vi "WPI_CANJaguar_GetPID.vi"(0 "CAN Jaguar Ref":T1={"DeviceStatus"={"status"=FALSE, "code"=0, "source"=""}, "Type"=enum."PWM", "PWM"={"PWM Channel"=enum."PWM 1", "DeadBand"={"Name"="", "maxPositivePwm"=0, "minPositivePwm"=0, "centerPwm"=0, "maxNegativePwm"=0, "minNegativePwm"=0, "angularRange"=0}}, "CAN"={"Device Number"=0, "SetOutput VI Ref"=variant(enum8{"Percent VBus", "Current", "Speed", "Position", "Voltage"} enum."Percent VBus"), "GetOutput VI Ref"=variant(refnum<k1> refnum), "Enable VI Ref"=variant(dbl 12.0), "Disable VI Ref"=variant(enum8{"Percent VBus", "Speed", "Position", "Slave", "Unchanged / Invalid", "Voltage Compensation", "Current", "Motion Profile"} enum."Percent VBus"), "Data"=variant}, "Invert"=FALSE}, 11 "error in (no error)":errorcluster) -> (4 "CAN Jaguar Ref":T1={"DeviceStatus"={"status"=FALSE, "code"=0, "source"=""}, "Type"=enum."PWM", "PWM"={"PWM Channel"=enum."PWM 1", "DeadBand"={"Name"="", "maxPositivePwm"=0, "minPositivePwm"=0, "centerPwm"=0, "maxNegativePwm"=0, "minNegativePwm"=0, "angularRange"=0}}, "CAN"={"Device Number"=0, "SetOutput VI Ref"=variant(enum8{"Percent VBus", "Current", "Speed", "Position", "Voltage"} enum."Percent VBus"), "GetOutput VI Ref"=variant(refnum<k1> refnum), "Enable VI Ref"=variant(dbl 12.0), "Disable VI Ref"=variant(enum8{"Percent VBus", "Speed", "Position", "Slave", "Unchanged / Invalid", "Voltage Compensation", "Current", "Motion Profile"} enum."Percent VBus"), "Data"=variant}, "Invert"=FALSE}, 6 "P":dbl, 8 "I":dbl, 10 "D":dbl, 15 "error out":errorcluster)   [LabVIEW 2016]
doc: "Get the PID constants that are being used by the active controller on the Jaguar.\n\nThis VI only applies in <B>Current</B>, <B>Position</B>, and <B>Speed</B> modes."
uses:
  <vilib>/Rock Robotics/WPI/MotorControl/WPI_MotorControlDeviceRef.ctl
  <vilib>/Rock Robotics/WPI/MotorControl/WPI_MotorControlType.ctl
  <vilib>/Rock Robotics/SystemInterfaces/DIO/FPGA_DIOPWMChannel.ctl
  <vilib>/Rock Robotics/WPI/PWM/WPI_PWMDeadband.ctl
  <vilib>/Rock Robotics/WPI/ThirdParty/CanMotor/CAN Jaguar/SubVIs/WPI_CANJaguar_RefNumData.ctl
  <vilib>/Rock Robotics/WPI/ThirdParty/CanMotor/CAN Jaguar/SubVIs/WPI_CANJaguar_ControlMode.ctl
  <vilib>/Rock Robotics/WPI/ThirdParty/CanMotor/CAN Jaguar/SubVIs/WPI_CAN_MotorMessageIDs.ctl
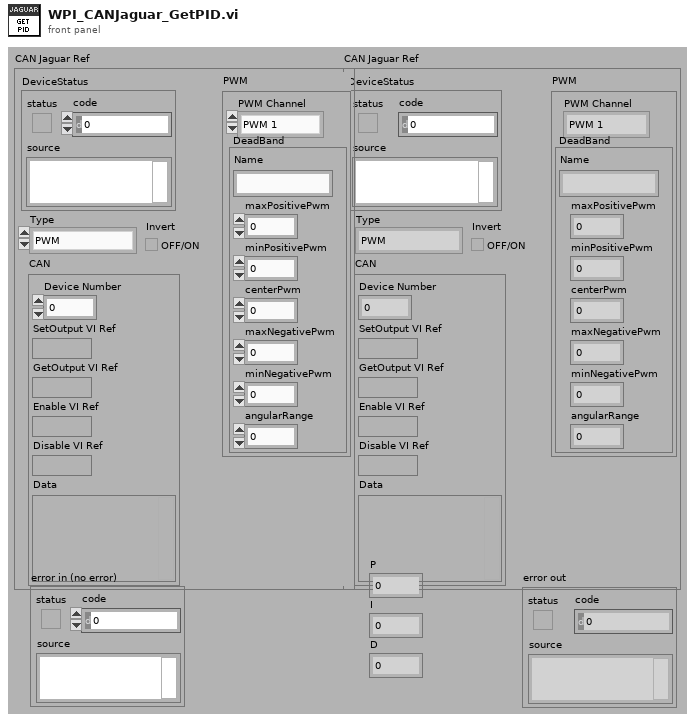
[diagram p1: front panel]
types:
  T1 = typedef "WPI_MotorControlDeviceRef.ctl" = cluster{"DeviceStatus":errorcluster, "Type":T2, "PWM":cluster{"PWM Channel":T3, "DeadBand":T4}, "CAN":cluster{"Device Number":u8, "SetOutput VI Ref":variant, "GetOutput VI Ref":variant, "Enable VI Ref":variant, "Disable VI Ref":variant, "Data":variant}, "Invert":bool}
  T2 = typedef "WPI_MotorControlType.ctl" = enum16{"PWM", "CAN"}
  T3 = typedef "FPGA_DIOPWMChannel.ctl" = enum8{"PWM 0", "PWM 1", "PWM 2", "PWM 3", "PWM 4", "PWM 5", "PWM 6", "PWM 7", "PWM 8", "PWM 9", "PWM MXP 0", "PWM MXP 1", "PWM MXP 2", "PWM MXP 3", "PWM MXP 4", "PWM MXP 5", "PWM MXP 6", "PWM MXP 7", "PWM MXP 8", "PWM MXP 9", "Invalid"}
  T4 = typedef "WPI_PWMDeadband.ctl" = cluster{"Name":string, "maxPositivePwm":i32, "minPositivePwm":i32, "centerPwm":i32, "maxNegativePwm":i32, "minNegativePwm":i32, "angularRange":u16}
  T5 = typedef "WPI_CANJaguar_RefNumData.ctl" = cluster{"CAN.Max Vout":dbl, "Control Mode":T6, "semaphore":T7}
  T6 = typedef "WPI_CANJaguar_ControlMode.ctl" = enum8{"Percent VBus", "Current", "Speed", "Position", "Voltage"}
  T7 = typedef "Semaphore RefNum" = refnum<k1>
  T8 = typedef "WPI_CAN_MotorMessageIDs.ctl" = u32
  T9 = enum16{"big-endian, network order", "native, host order", "little-endian"}
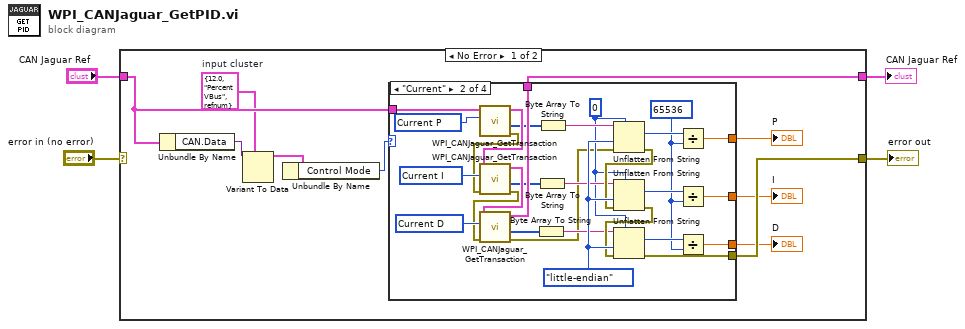
[diagram p0: block diagram]
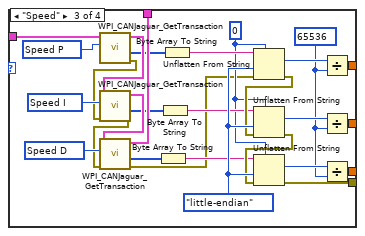
[diagram p3: hidden frame]
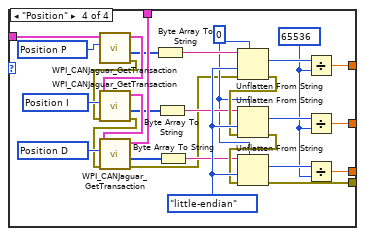
[diagram p4: hidden frame]
diagram:
  n1 = case shown="No Error" "error in (no error)" {
    selector: "error in (no error)" -> [_ w100]
    tunnel: [w9 w101] -> w4
    tunnel: "CAN Jaguar Ref" -> [w10 w101]
    tunnel: [w14 w100] -> w2
    frame No Error {
      w7 = T5 {"CAN.Max Vout"=12.0, "Control Mode"=enum."Percent VBus", "semaphore"=refnum}  # input cluster
      n2 = Unbundle By Name(w10) -> ("CAN.Data"=w8:variant)
      n3 = Variant To Data(type=w7, Variant=w8) -> (data=w6:T5)  [unwired: 1 in, 1 out]
      n4 = Unbundle By Name(w6) -> ("Control Mode"=w5:T6)
      n5 = case shown="\"Current\"" w5 {
        tunnel: [_ w34 w62 w90] -> w13
        tunnel: [_ w36 w64 w92] -> w14
        tunnel: [_ w32 w60 w88] -> w12
        tunnel: [_ w30 w58 w86] -> w11
        tunnel: w10 -> [w15 w28 w56 w84]
        tunnel: [w15 w21 w50 w78] -> w9
        frame Default {
        }
        frame "Current" {
          w29 = 65536 ("y")
          w26 = T8 33689856 items=["Volt Enable"=33685504, "Volt Disable"=33685568, "Volt Set"=33685632, "Volt Set Ramp"=33685696, "Speed Enable"=33686528, "Speed Disable"=33686592, "Speed Set"=33686656, "Speed P"=33686720, "Speed I"=33686784, "Speed D"=33686848, "Speed Ref"=33686912, "Volt Comp Enable"=33687552, "Volt Comp Disable"=33687616, "Volt Comp Set"=33687680, "Volt Comp In Ramp"=33687744, "Volt Comp Comp Ramp"=33687808, "Position Enable"=33688576, "Position Disable"=33688640, "Position Set"=33688704, "Position P"=33688768, "Position I"=33688832, "Position D"=33688896, "Position Ref"=33688960, "Current Enable"=33689600, "Current Disable"=33689664, "Current Set"=33689728, "Current P"=33689792, "Current I"=33689856, "Current D"=33689920, "Status Percent VBus"=33690624, "Status VBus"=33690688, "Status Current"=33690752, "Status Temp"=33690816, "Status Position"=33690880, "Status Speed"=33690944, "Status Limit"=33691008, "Status Fault"=33691072, "Status Power"=33691136, "Status Control Mode"=33691200, "Status VOut"=33691264, "Config Num Brushes"=33692672, "Config Encoder Lines"=33692736, "Config Pot Turns"=33692800, "Config Brake Coast"=33692864, "Config Limit Mode"=33692928, "Config Limit Fwd"=33692992, "Config Limit Rev"=33693056, "Config Max VOut"=33693120, "Config Fault Time"=33693184, "Motor Ack"=33693696] ("CAN Motor Message IDs")
          w24 = T8 33689920 items=["Volt Enable"=33685504, "Volt Disable"=33685568, "Volt Set"=33685632, "Volt Set Ramp"=33685696, "Speed Enable"=33686528, "Speed Disable"=33686592, "Speed Set"=33686656, "Speed P"=33686720, "Speed I"=33686784, "Speed D"=33686848, "Speed Ref"=33686912, "Volt Comp Enable"=33687552, "Volt Comp Disable"=33687616, "Volt Comp Set"=33687680, "Volt Comp In Ramp"=33687744, "Volt Comp Comp Ramp"=33687808, "Position Enable"=33688576, "Position Disable"=33688640, "Position Set"=33688704, "Position P"=33688768, "Position I"=33688832, "Position D"=33688896, "Position Ref"=33688960, "Current Enable"=33689600, "Current Disable"=33689664, "Current Set"=33689728, "Current P"=33689792, "Current I"=33689856, "Current D"=33689920, "Status Percent VBus"=33690624, "Status VBus"=33690688, "Status Current"=33690752, "Status Temp"=33690816, "Status Position"=33690880, "Status Speed"=33690944, "Status Limit"=33691008, "Status Fault"=33691072, "Status Power"=33691136, "Status Control Mode"=33691200, "Status VOut"=33691264, "Config Num Brushes"=33692672, "Config Encoder Lines"=33692736, "Config Pot Turns"=33692800, "Config Brake Coast"=33692864, "Config Limit Mode"=33692928, "Config Limit Fwd"=33692992, "Config Limit Rev"=33693056, "Config Max VOut"=33693120, "Config Fault Time"=33693184, "Motor Ack"=33693696] ("CAN Motor Message IDs")
          w37 = 0 ("Voltage")
          w27 = T8 33689792 items=["Volt Enable"=33685504, "Volt Disable"=33685568, "Volt Set"=33685632, "Volt Set Ramp"=33685696, "Speed Enable"=33686528, "Speed Disable"=33686592, "Speed Set"=33686656, "Speed P"=33686720, "Speed I"=33686784, "Speed D"=33686848, "Speed Ref"=33686912, "Volt Comp Enable"=33687552, "Volt Comp Disable"=33687616, "Volt Comp Set"=33687680, "Volt Comp In Ramp"=33687744, "Volt Comp Comp Ramp"=33687808, "Position Enable"=33688576, "Position Disable"=33688640, "Position Set"=33688704, "Position P"=33688768, "Position I"=33688832, "Position D"=33688896, "Position Ref"=33688960, "Current Enable"=33689600, "Current Disable"=33689664, "Current Set"=33689728, "Current P"=33689792, "Current I"=33689856, "Current D"=33689920, "Status Percent VBus"=33690624, "Status VBus"=33690688, "Status Current"=33690752, "Status Temp"=33690816, "Status Position"=33690880, "Status Speed"=33690944, "Status Limit"=33691008, "Status Fault"=33691072, "Status Power"=33691136, "Status Control Mode"=33691200, "Status VOut"=33691264, "Config Num Brushes"=33692672, "Config Encoder Lines"=33692736, "Config Pot Turns"=33692800, "Config Brake Coast"=33692864, "Config Limit Mode"=33692928, "Config Limit Fwd"=33692992, "Config Limit Rev"=33693056, "Config Max VOut"=33693120, "Config Fault Time"=33693184, "Motor Ack"=33693696] ("CAN Motor Message IDs")
          w42 = T9."little-endian" ("byte order (0:big-endian, network order)")
          n6 = call <vilib>:"WPI_CANJaguar_GetTransaction.vi"("Message ID"=w27, "CAN Jaguar Ref"=w28) -> ("error out"=w17:errorcluster, "Data Out"=w18:u8[], "CAN Jaguar Ref Out"=w25:T1)  [unwired: 1 in, 6 out]
          n7 = call <vilib>:"WPI_CANJaguar_GetTransaction.vi"("error in"=w17, "Message ID"=w26, "CAN Jaguar Ref"=w25) -> ("error out"=w16:errorcluster, "Data Out"=w19:u8[], "CAN Jaguar Ref Out"=w23:T1)  [unwired: 6 out]
          n8 = call <vilib>:"WPI_CANJaguar_GetTransaction.vi"("error in"=w16, "Message ID"=w24, "CAN Jaguar Ref"=w23) -> ("error out"=w22:errorcluster, "Data Out"=w20:u8[], "CAN Jaguar Ref Out"=w21:T1)  [unwired: 6 out]
          n9 = Byte Array To String(unsigned byte array=w20) -> (string=w38:string)
          n10 = Byte Array To String(unsigned byte array=w19) -> (string=w39:string)
          n11 = Byte Array To String(unsigned byte array=w18) -> (string=w43:string)
          n12 = Unflatten From String(type=w37, binary string=w43, byte order (0:big-endian, network order)=w42, error in (no error)=w22) -> (value=w35:i32, error out=w40:errorcluster)  [unwired: 2 out]
          n13 = Unflatten From String(type=w37, binary string=w39, byte order (0:big-endian, network order)=w42, error in (no error)=w40) -> (value=w33:i32, error out=w41:errorcluster)  [unwired: 2 out]
          n14 = Unflatten From String(type=w37, binary string=w38, byte order (0:big-endian, network order)=w42, error in (no error)=w41) -> (value=w31:i32, error out=w36:errorcluster)  [unwired: 2 out]
          n15 = Divide(x=w35, y=w29) -> (x/y=w34:dbl)
          n16 = Divide(x=w33, y=w29) -> (x/y=w32:dbl)
          n17 = Divide(x=w31, y=w29) -> (x/y=w30:dbl)
        }
        frame "Speed" {
          w57 = 65536 ("y")
          w54 = T8 33686784 items=["Volt Enable"=33685504, "Volt Disable"=33685568, "Volt Set"=33685632, "Volt Set Ramp"=33685696, "Speed Enable"=33686528, "Speed Disable"=33686592, "Speed Set"=33686656, "Speed P"=33686720, "Speed I"=33686784, "Speed D"=33686848, "Speed Ref"=33686912, "Volt Comp Enable"=33687552, "Volt Comp Disable"=33687616, "Volt Comp Set"=33687680, "Volt Comp In Ramp"=33687744, "Volt Comp Comp Ramp"=33687808, "Position Enable"=33688576, "Position Disable"=33688640, "Position Set"=33688704, "Position P"=33688768, "Position I"=33688832, "Position D"=33688896, "Position Ref"=33688960, "Current Enable"=33689600, "Current Disable"=33689664, "Current Set"=33689728, "Current P"=33689792, "Current I"=33689856, "Current D"=33689920, "Status Percent VBus"=33690624, "Status VBus"=33690688, "Status Current"=33690752, "Status Temp"=33690816, "Status Position"=33690880, "Status Speed"=33690944, "Status Limit"=33691008, "Status Fault"=33691072, "Status Power"=33691136, "Status Control Mode"=33691200, "Status VOut"=33691264, "Config Num Brushes"=33692672, "Config Encoder Lines"=33692736, "Config Pot Turns"=33692800, "Config Brake Coast"=33692864, "Config Limit Mode"=33692928, "Config Limit Fwd"=33692992, "Config Limit Rev"=33693056, "Config Max VOut"=33693120, "Config Fault Time"=33693184, "Motor Ack"=33693696] ("CAN Motor Message IDs")
          w51 = T8 33686848 items=["Volt Enable"=33685504, "Volt Disable"=33685568, "Volt Set"=33685632, "Volt Set Ramp"=33685696, "Speed Enable"=33686528, "Speed Disable"=33686592, "Speed Set"=33686656, "Speed P"=33686720, "Speed I"=33686784, "Speed D"=33686848, "Speed Ref"=33686912, "Volt Comp Enable"=33687552, "Volt Comp Disable"=33687616, "Volt Comp Set"=33687680, "Volt Comp In Ramp"=33687744, "Volt Comp Comp Ramp"=33687808, "Position Enable"=33688576, "Position Disable"=33688640, "Position Set"=33688704, "Position P"=33688768, "Position I"=33688832, "Position D"=33688896, "Position Ref"=33688960, "Current Enable"=33689600, "Current Disable"=33689664, "Current Set"=33689728, "Current P"=33689792, "Current I"=33689856, "Current D"=33689920, "Status Percent VBus"=33690624, "Status VBus"=33690688, "Status Current"=33690752, "Status Temp"=33690816, "Status Position"=33690880, "Status Speed"=33690944, "Status Limit"=33691008, "Status Fault"=33691072, "Status Power"=33691136, "Status Control Mode"=33691200, "Status VOut"=33691264, "Config Num Brushes"=33692672, "Config Encoder Lines"=33692736, "Config Pot Turns"=33692800, "Config Brake Coast"=33692864, "Config Limit Mode"=33692928, "Config Limit Fwd"=33692992, "Config Limit Rev"=33693056, "Config Max VOut"=33693120, "Config Fault Time"=33693184, "Motor Ack"=33693696] ("CAN Motor Message IDs")
          w65 = 0 ("Voltage")
          w55 = T8 33686720 items=["Volt Enable"=33685504, "Volt Disable"=33685568, "Volt Set"=33685632, "Volt Set Ramp"=33685696, "Speed Enable"=33686528, "Speed Disable"=33686592, "Speed Set"=33686656, "Speed P"=33686720, "Speed I"=33686784, "Speed D"=33686848, "Speed Ref"=33686912, "Volt Comp Enable"=33687552, "Volt Comp Disable"=33687616, "Volt Comp Set"=33687680, "Volt Comp In Ramp"=33687744, "Volt Comp Comp Ramp"=33687808, "Position Enable"=33688576, "Position Disable"=33688640, "Position Set"=33688704, "Position P"=33688768, "Position I"=33688832, "Position D"=33688896, "Position Ref"=33688960, "Current Enable"=33689600, "Current Disable"=33689664, "Current Set"=33689728, "Current P"=33689792, "Current I"=33689856, "Current D"=33689920, "Status Percent VBus"=33690624, "Status VBus"=33690688, "Status Current"=33690752, "Status Temp"=33690816, "Status Position"=33690880, "Status Speed"=33690944, "Status Limit"=33691008, "Status Fault"=33691072, "Status Power"=33691136, "Status Control Mode"=33691200, "Status VOut"=33691264, "Config Num Brushes"=33692672, "Config Encoder Lines"=33692736, "Config Pot Turns"=33692800, "Config Brake Coast"=33692864, "Config Limit Mode"=33692928, "Config Limit Fwd"=33692992, "Config Limit Rev"=33693056, "Config Max VOut"=33693120, "Config Fault Time"=33693184, "Motor Ack"=33693696] ("CAN Motor Message IDs")
          w70 = T9."little-endian" ("byte order (0:big-endian, network order)")
          n18 = call <vilib>:"WPI_CANJaguar_GetTransaction.vi"("Message ID"=w55, "CAN Jaguar Ref"=w56) -> ("error out"=w44:errorcluster, "Data Out"=w48:u8[], "CAN Jaguar Ref Out"=w53:T1)  [unwired: 1 in, 6 out]
          n19 = call <vilib>:"WPI_CANJaguar_GetTransaction.vi"("error in"=w44, "Message ID"=w54, "CAN Jaguar Ref"=w53) -> ("error out"=w45:errorcluster, "Data Out"=w47:u8[], "CAN Jaguar Ref Out"=w52:T1)  [unwired: 6 out]
          n20 = call <vilib>:"WPI_CANJaguar_GetTransaction.vi"("error in"=w45, "Message ID"=w51, "CAN Jaguar Ref"=w52) -> ("error out"=w49:errorcluster, "Data Out"=w46:u8[], "CAN Jaguar Ref Out"=w50:T1)  [unwired: 6 out]
          n21 = Byte Array To String(unsigned byte array=w46) -> (string=w66:string)
          n22 = Byte Array To String(unsigned byte array=w47) -> (string=w67:string)
          n23 = Byte Array To String(unsigned byte array=w48) -> (string=w71:string)
          n24 = Unflatten From String(type=w65, binary string=w71, byte order (0:big-endian, network order)=w70, error in (no error)=w49) -> (value=w63:i32, error out=w68:errorcluster)  [unwired: 2 out]
          n25 = Unflatten From String(type=w65, binary string=w67, byte order (0:big-endian, network order)=w70, error in (no error)=w68) -> (value=w61:i32, error out=w69:errorcluster)  [unwired: 2 out]
          n26 = Unflatten From String(type=w65, binary string=w66, byte order (0:big-endian, network order)=w70, error in (no error)=w69) -> (value=w59:i32, error out=w64:errorcluster)  [unwired: 2 out]
          n27 = Divide(x=w63, y=w57) -> (x/y=w62:dbl)
          n28 = Divide(x=w61, y=w57) -> (x/y=w60:dbl)
          n29 = Divide(x=w59, y=w57) -> (x/y=w58:dbl)
        }
        frame "Position" {
          w85 = 65536 ("y")
          w81 = T8 33688832 items=["Volt Enable"=33685504, "Volt Disable"=33685568, "Volt Set"=33685632, "Volt Set Ramp"=33685696, "Speed Enable"=33686528, "Speed Disable"=33686592, "Speed Set"=33686656, "Speed P"=33686720, "Speed I"=33686784, "Speed D"=33686848, "Speed Ref"=33686912, "Volt Comp Enable"=33687552, "Volt Comp Disable"=33687616, "Volt Comp Set"=33687680, "Volt Comp In Ramp"=33687744, "Volt Comp Comp Ramp"=33687808, "Position Enable"=33688576, "Position Disable"=33688640, "Position Set"=33688704, "Position P"=33688768, "Position I"=33688832, "Position D"=33688896, "Position Ref"=33688960, "Current Enable"=33689600, "Current Disable"=33689664, "Current Set"=33689728, "Current P"=33689792, "Current I"=33689856, "Current D"=33689920, "Status Percent VBus"=33690624, "Status VBus"=33690688, "Status Current"=33690752, "Status Temp"=33690816, "Status Position"=33690880, "Status Speed"=33690944, "Status Limit"=33691008, "Status Fault"=33691072, "Status Power"=33691136, "Status Control Mode"=33691200, "Status VOut"=33691264, "Config Num Brushes"=33692672, "Config Encoder Lines"=33692736, "Config Pot Turns"=33692800, "Config Brake Coast"=33692864, "Config Limit Mode"=33692928, "Config Limit Fwd"=33692992, "Config Limit Rev"=33693056, "Config Max VOut"=33693120, "Config Fault Time"=33693184, "Motor Ack"=33693696] ("CAN Motor Message IDs")
          w82 = T8 33688896 items=["Volt Enable"=33685504, "Volt Disable"=33685568, "Volt Set"=33685632, "Volt Set Ramp"=33685696, "Speed Enable"=33686528, "Speed Disable"=33686592, "Speed Set"=33686656, "Speed P"=33686720, "Speed I"=33686784, "Speed D"=33686848, "Speed Ref"=33686912, "Volt Comp Enable"=33687552, "Volt Comp Disable"=33687616, "Volt Comp Set"=33687680, "Volt Comp In Ramp"=33687744, "Volt Comp Comp Ramp"=33687808, "Position Enable"=33688576, "Position Disable"=33688640, "Position Set"=33688704, "Position P"=33688768, "Position I"=33688832, "Position D"=33688896, "Position Ref"=33688960, "Current Enable"=33689600, "Current Disable"=33689664, "Current Set"=33689728, "Current P"=33689792, "Current I"=33689856, "Current D"=33689920, "Status Percent VBus"=33690624, "Status VBus"=33690688, "Status Current"=33690752, "Status Temp"=33690816, "Status Position"=33690880, "Status Speed"=33690944, "Status Limit"=33691008, "Status Fault"=33691072, "Status Power"=33691136, "Status Control Mode"=33691200, "Status VOut"=33691264, "Config Num Brushes"=33692672, "Config Encoder Lines"=33692736, "Config Pot Turns"=33692800, "Config Brake Coast"=33692864, "Config Limit Mode"=33692928, "Config Limit Fwd"=33692992, "Config Limit Rev"=33693056, "Config Max VOut"=33693120, "Config Fault Time"=33693184, "Motor Ack"=33693696] ("CAN Motor Message IDs")
          w93 = 0 ("Voltage")
          w83 = T8 33688768 items=["Volt Enable"=33685504, "Volt Disable"=33685568, "Volt Set"=33685632, "Volt Set Ramp"=33685696, "Speed Enable"=33686528, "Speed Disable"=33686592, "Speed Set"=33686656, "Speed P"=33686720, "Speed I"=33686784, "Speed D"=33686848, "Speed Ref"=33686912, "Volt Comp Enable"=33687552, "Volt Comp Disable"=33687616, "Volt Comp Set"=33687680, "Volt Comp In Ramp"=33687744, "Volt Comp Comp Ramp"=33687808, "Position Enable"=33688576, "Position Disable"=33688640, "Position Set"=33688704, "Position P"=33688768, "Position I"=33688832, "Position D"=33688896, "Position Ref"=33688960, "Current Enable"=33689600, "Current Disable"=33689664, "Current Set"=33689728, "Current P"=33689792, "Current I"=33689856, "Current D"=33689920, "Status Percent VBus"=33690624, "Status VBus"=33690688, "Status Current"=33690752, "Status Temp"=33690816, "Status Position"=33690880, "Status Speed"=33690944, "Status Limit"=33691008, "Status Fault"=33691072, "Status Power"=33691136, "Status Control Mode"=33691200, "Status VOut"=33691264, "Config Num Brushes"=33692672, "Config Encoder Lines"=33692736, "Config Pot Turns"=33692800, "Config Brake Coast"=33692864, "Config Limit Mode"=33692928, "Config Limit Fwd"=33692992, "Config Limit Rev"=33693056, "Config Max VOut"=33693120, "Config Fault Time"=33693184, "Motor Ack"=33693696] ("CAN Motor Message IDs")
          w98 = T9."little-endian" ("byte order (0:big-endian, network order)")
          n30 = call <vilib>:"WPI_CANJaguar_GetTransaction.vi"("Message ID"=w83, "CAN Jaguar Ref"=w84) -> ("error out"=w72:errorcluster, "Data Out"=w74:u8[], "CAN Jaguar Ref Out"=w80:T1)  [unwired: 1 in, 6 out]
          n31 = call <vilib>:"WPI_CANJaguar_GetTransaction.vi"("error in"=w72, "Message ID"=w81, "CAN Jaguar Ref"=w80) -> ("error out"=w73:errorcluster, "Data Out"=w75:u8[], "CAN Jaguar Ref Out"=w79:T1)  [unwired: 6 out]
          n32 = call <vilib>:"WPI_CANJaguar_GetTransaction.vi"("error in"=w73, "Message ID"=w82, "CAN Jaguar Ref"=w79) -> ("error out"=w77:errorcluster, "Data Out"=w76:u8[], "CAN Jaguar Ref Out"=w78:T1)  [unwired: 6 out]
          n33 = Byte Array To String(unsigned byte array=w74) -> (string=w99:string)
          n34 = Byte Array To String(unsigned byte array=w75) -> (string=w95:string)
          n35 = Byte Array To String(unsigned byte array=w76) -> (string=w94:string)
          n36 = Unflatten From String(type=w93, binary string=w99, byte order (0:big-endian, network order)=w98, error in (no error)=w77) -> (value=w91:i32, error out=w96:errorcluster)  [unwired: 2 out]
          n37 = Unflatten From String(type=w93, binary string=w95, byte order (0:big-endian, network order)=w98, error in (no error)=w96) -> (value=w89:i32, error out=w97:errorcluster)  [unwired: 2 out]
          n38 = Unflatten From String(type=w93, binary string=w94, byte order (0:big-endian, network order)=w98, error in (no error)=w97) -> (value=w87:i32, error out=w92:errorcluster)  [unwired: 2 out]
          n39 = Divide(x=w91, y=w85) -> (x/y=w90:dbl)
          n40 = Divide(x=w89, y=w85) -> (x/y=w88:dbl)
          n41 = Divide(x=w87, y=w85) -> (x/y=w86:dbl)
        }
      }
      "P" <- w13
      "I" <- w12
      "D" <- w11
    }
    frame Error {
    }
  }
  "CAN Jaguar Ref" <- w4
  "error out" <- w2
